vi "genIOL_Insertion.vi"(11 "Arm ID Ind":i32) -> (0 "zVisTraj":dbl[](array[numeric]) format="%_6g", 1 "yVisTraj":dbl[](array[numeric]) format="%_6g", 2 "xVisTraj":dbl[](array[numeric]) format="%_6g")   [LabVIEW 2016]
uses:
  <vilib>/Math Plots/3D Math Plots/3D Scatter/3D Scatter XCtrl/3D Scatter.xctl
  <vilib>/Math Plots/3D Math Plots/3D Scatter/3D Scatter Datatype/Public/Plot Helper (Vector).vi
  <vilib>/Analysis/NI_AALBase.lvlib
  <vilib>/Analysis/1siggen.llb/Ramp Pattern by Samples.vi
  <vilib>/gmath/NI_Gmath.lvlib
  Subsystems/Global Variables.vi
  <vilib>/Math Plots/3D Math Plots/3D Scatter/3D Scatter Datatype/3D Scatter Datatype.lvclass
panel:
  out "traj operational space":dbl[][](array[numeric])
  out "ind2":dbl
  out "ind1":dbl
  out "joint angles":dbl[][](array[numeric])
  in  "index":i32=200
  in  "PC path":path=path "D:/IRISSoft LV2016 beta/Host Demo/ThorlabsData/Eye1/VSCAN_0003.raw"
  in  "Iris path":path=path "D:/IRISSoft LV2016 beta/Host Demo/ThorlabsData/Eye1/VSCAN_0002.raw"
  out "Incision point":dbl[](array[numeric])
  out "Implement Injection Plot":refnum<class "3D Plot Datatype.lvclass">[](xcontrol)
  out "Implement joint angles":dbl[][](graph)
  out "min dist":dbl
  out "Actual Injection Plot":refnum<class "3D Plot Datatype.lvclass">[](xcontrol)
  out "End manual joint":dbl[](array[numeric])
  out "Start manual joint":dbl[](array[numeric])
  out "Planed joint angles":dbl[][](graph)
  out "Whole joint angles":dbl[][](graph)
  out "traj":dbl[][](array[numeric])
  out "ind":dbl
  out "Offset":dbl[][](array[numeric])
  out "Incision point index":dbl
  out "Planed Injection Plot":refnum<class "3D Plot Datatype.lvclass">[](xcontrol)
  out "current loop #":dbl
  out "x coordinates size 3":dbl
  out "x coordinates size 2":dbl
  out "x coordinates size":dbl
  out "x coordinates":dbl[](array[numeric])
  out "z coordinates":dbl[](array[numeric]) format="%#_13g"
  out "y coordinates":dbl[](array[numeric]) format="%#_13g"
  out "x coodi 2nd":dbl[](array[numeric]) format="%#_13g"
  in  "Total Time":dbl=60.0
  in  "Tip out Posit":dbl[](array[numeric])=[0.0, 0.0, 0.0] caption="Position [mm]" format="%#.3f"
  in  "Cycle Time [sec]":dbl[](array[numeric])=[60.0, 90.0, 120.0]
  in  "Sampling Rate [Hz]":i32=1000
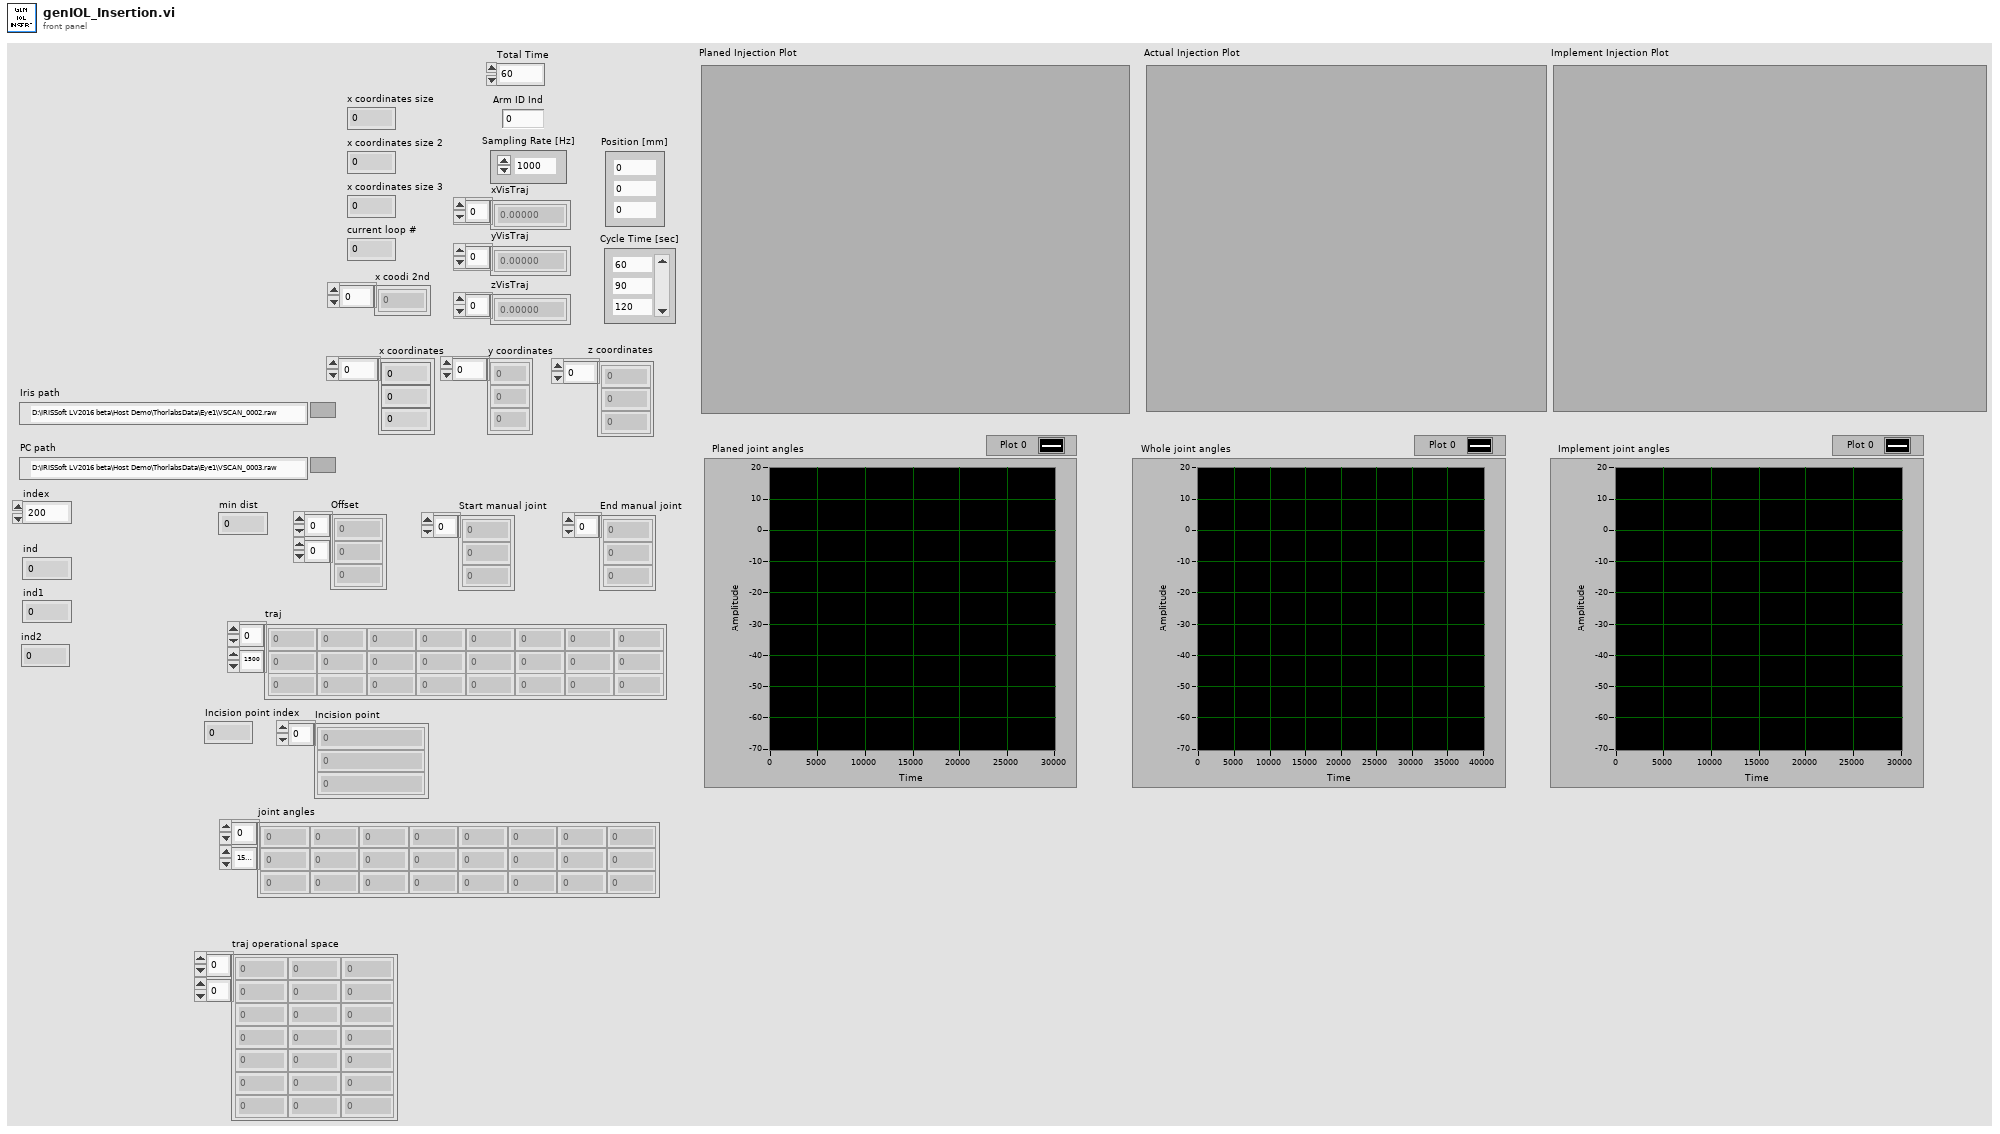
[diagram p1: front panel]
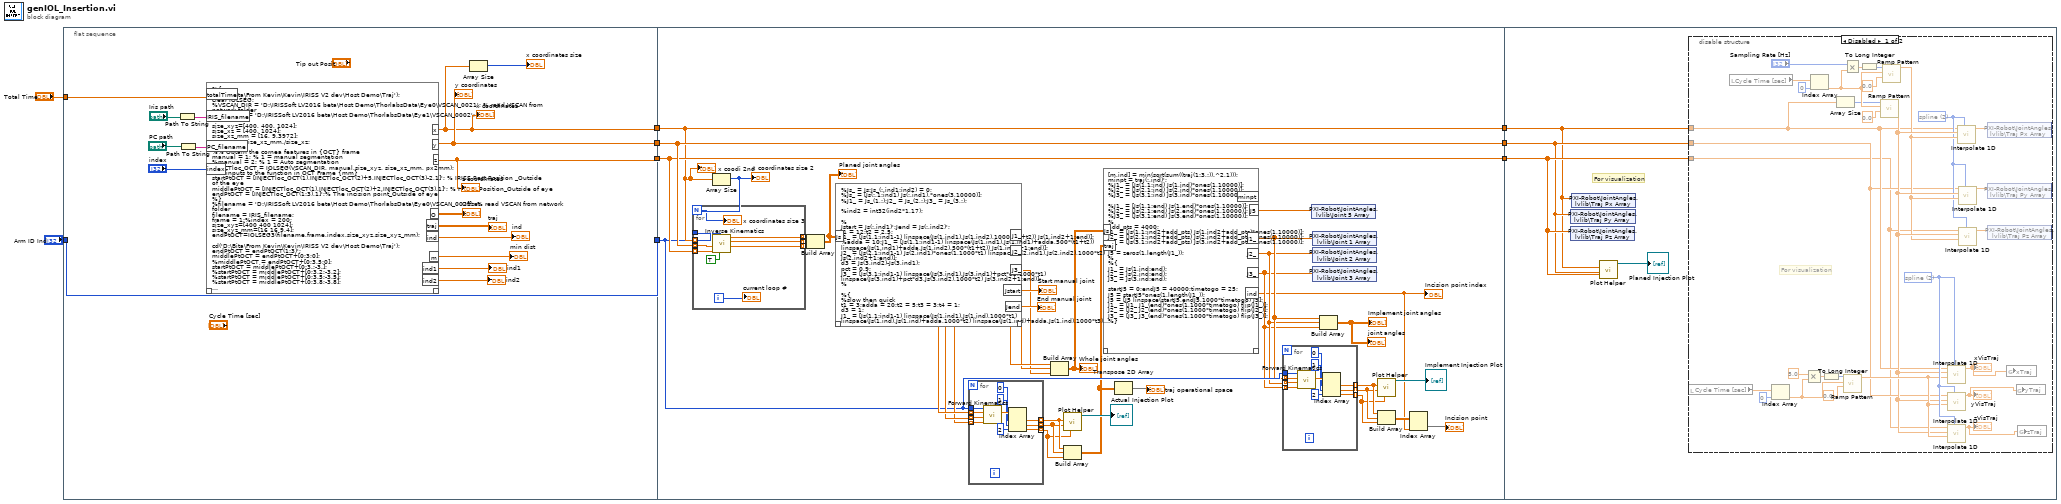
[diagram p0: block diagram]
diagram:
  n1 = flat-sequence {
    tunnel: "Arm ID Ind" -> [w26]
    tunnel: [w26] -> w8
    tunnel: [w22] -> w4
    tunnel: [w24] -> w3
    tunnel: [w23] -> w2
    tunnel: "Total Time" -> [w25]
    tunnel: w8 -> [w37]
    tunnel: [w57] -> w7
    tunnel: [w59] -> w6
    tunnel: [w58] -> w5
    tunnel: w4 -> [w57]
    tunnel: w3 -> [w59]
    tunnel: w2 -> [w58]
    tunnel: w7 -> [w92]
    tunnel: w6 -> [w93]
    tunnel: w5 -> [w94]
    frame #0 {
      n2 = Path To String(path="Iris path") -> (string=w15:string)
      n3 = Path To String(path="PC path") -> (string=w16:string)
      n4 = script code="%{\ncd('D:\\Bita\\From Kevin\\Kevin\\IRISS V2 dev\\Host Demo\\Traj');\nclear IOLSEG;\n%VSCAN_DIR = 'D:\\IRISSoft LV2016 beta\\Host Demo\\ThorlabsData\\Eye0\\VSCAN_0021'; % read VSCAN from network folder \nVSCAN_DIR = 'D:\\IRISSoft LV2016 beta\\Host Demo\\ThorlabsData\\Eye1\\VSCAN_0002';\n\nsize_xyz=[400, 400, 1024];\nsize_xz = [400, 1024]; \nsize_xz_mm = [16, 9.3972]; \npx2mm = size_xz_mm./size_xz; \n    \n%% Obtain the cornea features in {OCT} frame\nmanual = 1; % 1 = manual segmentation\n%manual = 2; % 1 = Auto segmentation\nINJECTloc_OCT = IOLSEG(VSCAN_DIR, manual,size_xyz, size_xz_mm, px2mm);\n%% inputs to the function in OCT Frame {mm}\nstartPtOCT = [INJECTloc_OCT(1),INJECTloc_OCT(2)+5,INJECTloc_OCT(3)-2,1]'; % IRISS Rest Position _Outside of the eye\nmiddlePtOCT = [INJECTloc_OCT(1),INJECTloc_OCT(2)+2,INJECTloc_OCT(3),1]'; % Home Position_Outside of eye\nendPtOCT = [INJECTloc_OCT(1:3),1]';% The incision point_Outside of eye\n%}\n%filename = 'D:\\IRISSoft LV2016 beta\\Host Demo\\ThorlabsData\\Eye0\\VSCAN_0021'; % read VSCAN from network folder \nfilename = IRIS_filename;\nframe = 1;%index = 200;\nsize_xyz=[400 400 1024];\nsize_xyz_mm=[16 16 9.4];\nendPtOCT=IOLSEG3(filename,frame,index,size_xyz,size_xyz_mm);\n\ncd('D:\\Bita\\From Kevin\\Kevin\\IRISS V2 dev\\Host Demo\\Traj');\nendPtOCT = endPtOCT(1:3)';\nmiddlePtOCT = endPtOCT+[0;3;0];\n%middlePtOCT = endPtOCT+[0;3.5;0];\nstartPtOCT = middlePtOCT+[0;3.;-3.];\n%startPtOCT = middlePtOCT+[0;3.2;-3.2];\n%startPtOCT = middlePtOCT+[0;3.5;-3.5];\n%startPtOCT = middlePtOCT+[0;3.8;-3.8];\n\n%middlePtOCT = endPtOCT+[0;-3;0];\n%startPtOCT = middlePtOCT+[0;-3.8;-3.8];\n\n%IRIS_filename = 'D:\\IRISSoft LV2016 beta\\Host Demo\\ThorlabsData\\Eye0\\VSCAN_0021.raw';\n%PC_filename = 'D:\\IRISSoft LV2016 beta\\Host Demo\\ThorlabsData\\Eye0\\VSCAN_0022.raw';\n%OCT_offset = 7; %OCT_offset = 0;\n%IRIS_filename = 'D:\\IRISSoft LV2016 beta\\Host Demo\\ThorlabsData\\Eye1\\VSCAN_0002.raw';\n%PC_filename = 'D:\\IRISSoft LV2016 beta\\Host Demo\\ThorlabsData\\Eye1\\VSCAN_0003.raw';\nOCT_offset = 13;\nspeed_scaler = 0.15;\n[tts,traj2,ind1,ind2]=IOL_injection_trajectory(startPtOCT,middlePtOCT,endPtOCT,IRIS_filename,PC_filename,OCT_offset,speed_scaler);\nTOI_file= 'D:\\IRISSoft LV2016 beta\\Host Demo\\TOI_static';\nfid_TOI = fopen(TOI_file,'r');\nTOI=fscanf(fid_TOI,'%f');\nTOI= reshape(TOI, [4 4])';\nfclose(fid_TOI);\n\nO = inv(TOI)*[endPtOCT;1];\n%{\ninit_X = 40;init_Y = 55;init_Z = 100;\ntime_to_go = norm(O(1:3))/.5;\nstage_X = linspace(init_X,init_X+O(1),1000*time_to_go);\nstage_Y = linspace(init_Y,init_Y+O(2),1000*time_to_go);\nstage_Z = linspace(init_Z,init_Z+O(3),1000*time_to_go);\n%}\n\nTOI2 = inv(TOI);TOI2(1:3,4) = TOI2(1:3,4)-O(1:3);\ntraj = TOI2*[traj2;ones(1,size(traj2,2))];\n%{\nTOI2_file= 'D:\\IRISSoft LV2016 beta\\Host Demo\\new_TOI.txt'\nfid_TOI2 = fopen(TOI2_file,'r');\nTOI2=fscanf(fid_TOI2,'%f');\nTOI2= reshape(TOI2, [4 4]);\nfclose(fid_TOI2);\ntraj = inv(TOI2)*[traj2;ones(1,size(traj2,2))];\n%}\n\nx = traj(1,:);y = traj(2,:);z = traj(3,:);\n[m,ind] = min(sqrt(sum((traj(1:3,:)).^2,1)));"("totalTime"=w25, "IRIS_filename"=w15, "PC_filename"=w16, "index"="index") -> ("x"=w22:dbl[], "y"=w24:dbl[], "z"=w23:dbl[], "O"=→"Offset":dbl[][], "ind"=→"ind":dbl, "traj"=→"traj":dbl[][], "ind1"=→"ind1":dbl, "ind2"=→"ind2":dbl, "m"=→"min dist":dbl)  [unwired: 1 in, 1 out]
      "y coordinates" <- w24
      "z coordinates" <- w23
      "x coordinates" <- w22
      n5 = Array Size(array=w22) -> (size(s)=→"x coordinates size":i32)
    }
    frame #1 {
      n6 = Array Size(array=w57) -> (size(s)=w56:i32)
      "x coordinates size 2" <- w56
      n7 = for {
        N: w56 -> [w86]
        tunnel: w37 -> [w87]
        tunnel: w57 -> [w91] mode=indexing
        tunnel: w59 -> [w90] mode=indexing
        tunnel: w58 -> [w89] mode=indexing
        tunnel: [w84] -> w54 mode=indexing
        tunnel: [w83] -> w53 mode=indexing
        tunnel: [w82] -> w55 mode=indexing
        i -> [w85]
        n8 = call "Inverse Kinematics.vi"("isToolTipInsideEye"=TRUE, "armID"=w87, "z"=w89, "y"=w90, "x"=w91) -> ("j3"=w83:dbl, "j2"=w84:dbl, "j1"=w82:dbl)  [unwired: 3 in, 1 out]
        "x coordinates size 3" <- w86
        "current loop #" <- w85
      }
      n9 = Build Array(w55, w54, w53) -> (w52:dbl[][])
      "Planed joint angles" <- w52
      n10 = script code="%Js_ = Js;Js_(:,ind1:ind2) = 0;\n%Js_ = [Js(:,1:ind1) Js(:,ind1).*ones(3,10000)];\n%J1_ = Js_(1,:);J2_ = Js_(2,:);J3_ = Js_(3,:);\n\n%ind2 = int32(ind2*1.17);\n\n%\nJstart = Js(:,ind1)';Jend = Js(:,ind2)';\nt1 = 12;t2 = 2.5;\nJ1_ = [Js(1,1:ind1-1) linspace(Js(1,ind1),Js(1,ind2),1000*(t1+t2)) Js(1,ind2+1:end)];\n%adda = 10;J1_ = [Js(1,1:ind1-1) linspace(Js(1,ind1),Js(1,ind1)+adda,500*(t1+t2)) linspace(Js(1,ind1)+adda,Js(1,ind2),500*(t1+t2)) Js(1,ind2+1:end)];\nJ2_ = [Js(2,1:ind1-1) Js(2,ind1)*ones(1,1000*t1) linspace(Js(2,ind1),Js(2,ind2),1000*t2) Js(2,ind2+1:end)];\nd3 = Js(3,ind2)-Js(3,ind1);\npct = 0.9;\nJ3_ = [Js(3,1:ind1-1) linspace(Js(3,ind1),Js(3,ind1)+pct*d3,1000*t1) linspace(Js(3,ind1)+pct*d3,Js(3,ind2),1000*t2) Js(3,ind2+1:end)];\n%\n\n%{\n%slow then quick\nt1 = 3;adda = 20;t2 = 5;t3 = 3;t4 = 1;\nd3 = 1;\nJ1_ = [Js(1,1:ind1-1) linspace(Js(1,ind1),Js(1,ind),1000*t1) linspace(Js(1,ind),Js(1,ind)+adda,1000*t2) linspace(Js(1,ind)+adda,Js(1,ind),1000*t3) linspace(Js(1,ind),Js(1,ind2),1000*t4)];\nJ2_ = [Js(2,1:ind1-1) linspace(Js(2,ind1),Js(2,ind),1000*t1) Js(2,ind)*ones(1,1000*(t2+t3)) linspace(Js(2,ind),Js(2,ind2),1000*t4)];\nJ3_ = [Js(3,1:ind1-1) linspace(Js(3,ind1),Js(3,ind),1000*t1) linspace(Js(3,ind),Js(3,ind)+d3,1000*t2) (Js(3,ind)+d3)*ones(1,1000*t3) linspace(Js(3,ind)+d3,Js(3,ind2),1000*t4)];\nlim_angle1 = -65;\nJ1_ = max(J1_,lim_angle1);\n%}\n%J1_ = [J1_(1:ind) J1_(ind)*ones(1,10000)];\n%J2_ = [J2_(1:ind) J2_(ind)*ones(1,10000)];\n%J3_ = [J3_(1:ind) J3_(ind)*ones(1,10000)];\n\n%startJ5 = 0;endJ5 = 40000;timetogo = 25;\n%J5 = startJ5*ones(1,length(J1_));\n%J5 = [J5 linspace(startJ5,endJ5,1000*timetogo) J5];\n%J1_ = [J1_ J1_(end)*ones(1,1000*timetogo) flip(J1_)];\n%J2_ = [J2_ J2_(end)*ones(1,1000*timetogo) flip(J2_)];\n%J3_ = [J3_ J3_(end)*ones(1,1000*timetogo) flip(J3_)];"("Js"=w52) -> ("J1_"=w49:dbl[], "J2_"=w48:dbl[], "J3_"=w47:dbl[], "Jstart"=→"Start manual joint":dbl[], "Jend"=→"End manual joint":dbl[])  [unwired: 1 in, 1 out]
      n11 = for {
        tunnel: w37 -> [w81]
        tunnel: w49 -> [w80] mode=indexing
        tunnel: w48 -> [w79] mode=indexing
        tunnel: w47 -> [w78] mode=indexing
        tunnel: [w73] -> w45 mode=indexing
        tunnel: [w72] -> w44 mode=indexing
        tunnel: [w71] -> w43 mode=indexing
        n12 = call "Forward Kinematics.vi"("j3"=w78, "j2"=w79, "j1"=w80, "armID"=w81) -> ("XYZ Out Array"=w77:dbl[])  [unwired: 7 in]
        n13 = Index Array(array=w77, index #1=0 ("index"), index #2=1 ("index"), index #3=2 ("index")) -> (element #1=w73:dbl, element #2=w72:dbl, element #3=w71:dbl)
      }
      n14 = Build Array(w49, w48, w47) -> (w36:dbl[][])
      "Whole joint angles" <- w36
      n15 = call-poly <vilib>:"Plot Helper.vi"("z vector"=w43, "y vector"=w44, "x vector"=w45) -> ("3D Plot lvclass Array out"=→"Actual Injection Plot":refnum<class "3D Plot Datatype.lvclass">[])  [unwired: 3 in, 5 out]
      n16 = Build Array(w45, w44, w43) -> (w27:dbl[][])
      n17 = script code="[m,ind] = min(sqrt(sum((traj(1:3,:)).^2,1)));\nminpt = traj(:,ind)';\n%J1_ = [Js(1,1:ind) Js(1,ind)*ones(1,10000)];\n%J2_ = [Js(2,1:ind) Js(2,ind)*ones(1,10000)];\n%J3_ = [Js(3,1:ind) Js(3,ind)*ones(1,10000)];\n\n%J1_ = [Js(1,1:end) Js(1,end)*ones(1,10000)];\n%J2_ = [Js(2,1:end) Js(2,end)*ones(1,10000)];\n%J3_ = [Js(3,1:end) Js(3,end)*ones(1,10000)];\n%\nadd_pts = 4000;\nJ1_ = [Js(1,1:ind2+add_pts) Js(1,ind2+add_pts)*ones(1,10000)];\nJ2_ = [Js(2,1:ind2+add_pts) Js(2,ind2+add_pts)*ones(1,10000)];\nJ3_ = [Js(3,1:ind2+add_pts) Js(3,ind2+add_pts)*ones(1,10000)];\n\nJ5 = zeros(1,length(J1_));\n%\n%{\nJ1_ = Js(1,ind:end);\nJ2_ = Js(2,ind:end);\nJ3_ = Js(3,ind:end);\n\nstartJ5 = 0;endJ5 = 40000;timetogo = 25;\nJ5 = startJ5*ones(1,length(J1_));\nJ5 = [J5 linspace(startJ5,endJ5,1000*timetogo) J5];\nJ1_ = [J1_ J1_(end)*ones(1,1000*timetogo) flip(J1_)];\nJ2_ = [J2_ J2_(end)*ones(1,1000*timetogo) flip(J2_)];\nJ3_ = [J3_ J3_(end)*ones(1,1000*timetogo) flip(J3_)];\n%}"("Js"=w36, "traj"=w27) -> ("J1_"=w35:dbl[], "J2_"=w34:dbl[], "J3_"=w33:dbl[], "ind"=w31:dbl, "J5"=w38:dbl[])  [unwired: 1 in, 2 out]
      "Incision point index" <- w31
      n18 = Transpose 2D Array(2D array=w27) -> (transposed array=→"traj operational space":dbl[][])
      n19 = for {
        tunnel: w37 -> [w70]
        tunnel: w35 -> [w69] mode=indexing
        tunnel: w34 -> [w68] mode=indexing
        tunnel: w33 -> [w67] mode=indexing
        tunnel: [w62] -> w41 mode=indexing
        tunnel: [w61] -> w40 mode=indexing
        tunnel: [w60] -> w39 mode=indexing
        n20 = call "Forward Kinematics.vi"("j3"=w67, "j2"=w68, "j1"=w69, "armID"=w70) -> ("XYZ Out Array"=w66:dbl[])  [unwired: 7 in]
        n21 = Index Array(array=w66, index #1=0 ("index"), index #2=1 ("index"), index #3=2 ("index")) -> (element #1=w62:dbl, element #2=w61:dbl, element #3=w60:dbl)
      }
      n22 = shared-variable "PXI-Robot\\JointAngles.lvlib\\Joint 5 Array"(w38) -> ()  [unwired: 1 in, 1 out]
      n23 = shared-variable "PXI-Robot\\JointAngles.lvlib\\Joint 1 Array"(w35) -> ()  [unwired: 1 in, 1 out]
      n24 = shared-variable "PXI-Robot\\JointAngles.lvlib\\Joint 2 Array"(w34) -> ()  [unwired: 1 in, 1 out]
      n25 = shared-variable "PXI-Robot\\JointAngles.lvlib\\Joint 3 Array"(w33) -> ()  [unwired: 1 in, 1 out]
      n26 = Build Array(w35, w34, w33) -> (→"Implement joint angles" →"joint angles":dbl[][])
      n27 = call-poly <vilib>:"Plot Helper.vi"("z vector"=w39, "y vector"=w40, "x vector"=w41) -> ("3D Plot lvclass Array out"=→"Implement Injection Plot":refnum<class "3D Plot Datatype.lvclass">[])  [unwired: 3 in, 5 out]
      n28 = Build Array(w41, w40, w39) -> (w32:dbl[][])
      n29 = Index Array(array=w32, index (col)=w31) -> (element=→"Incision point":dbl[])  [unwired: 1 in]
      "x coodi 2nd" <- w57
    }
    frame #2 {
      # "For visualization"
      n30 = shared-variable "PXI-Robot\\JointAngles.lvlib\\Traj Py Array"(w93) -> ()  [unwired: 1 in, 1 out]
      n31 = shared-variable "PXI-Robot\\JointAngles.lvlib\\Traj Pz Array"(w94) -> ()  [unwired: 1 in, 1 out]
      n32 = shared-variable "PXI-Robot\\JointAngles.lvlib\\Traj Px Array"(w92) -> ()  [unwired: 1 in, 1 out]
      n33 = call-poly <vilib>:"Plot Helper.vi"("z vector"=w94, "y vector"=w93, "x vector"=w92) -> ("3D Plot lvclass Array out"=→"Planed Injection Plot":refnum<class "3D Plot Datatype.lvclass">[])  [unwired: 3 in, 5 out]
      n34 = disable-structure shown="Disabled" {
        disable-tunnel: w92 -> [w101 _]
        disable-tunnel: w93 -> [w100 _]
        disable-tunnel: w94 -> [w99 _]
        frame Disabled {
          w113 = 2 items=["nearest", "linear", "spline", "cubic Hermite", "Lagrange"] ("method")
          w102 = 2 items=["nearest", "linear", "spline", "cubic Hermite", "Lagrange"] ("method")
          # "For visualization"
          n35 = local read "Cycle Time [sec]"() -> (w107:dbl[])
          n36 = local read "Cycle Time [sec]"() -> (w125:dbl[])
          n37 = Index Array(array=w107, index=0) -> (element=w108:dbl)
          n38 = Multiply(x=5.0, y=w108) -> (x*y=w110:dbl)
          n39 = Index Array(array=w125, index=0) -> (element=w118:dbl)
          n40 = To Long Integer(number=w110) -> (32bit integer=w111:i32)
          n41 = Array Size(array=w101) -> (size(s)=w117:i32)
          n42 = call-poly <vilib>:"Ramp Pattern.vi"("start"=0.0, "end"=w108, "samples"=w111) -> ("Ramp Pattern"=w105:dbl[])  [unwired: 7 in, 1 out]
          n43 = Multiply(x="Sampling Rate [Hz]", y=w118) -> (x*y=w121:dbl)
          n44 = To Long Integer(number=w121) -> (32bit integer=w122:i32)
          n45 = call-poly <vilib>:"Ramp Pattern.vi"("start"=0.0, "end"=w118, "samples"=w117) -> ("Ramp Pattern"=w104:dbl[])  [unwired: 7 in, 1 out]
          n46 = call-poly <vilib>:"Ramp Pattern.vi"("start"=0.0, "end"=w118, "samples"=w122) -> ("Ramp Pattern"=w103:dbl[])  [unwired: 7 in, 1 out]
          n47 = call <vilib>:"Interpolate 1D.vi"("method"=w113, "xi"=w105, "X"=w104, "Y"=w101) -> ("yi"=w96:dbl[])  [unwired: 5 in, 2 out]
          "xVisTraj" <- w96
          n48 = call <vilib>:"Interpolate 1D.vi"("method"=w113, "xi"=w105, "X"=w104, "Y"=w100) -> ("yi"=w97:dbl[])  [unwired: 5 in, 2 out]
          "yVisTraj" <- w97
          n49 = call <vilib>:"Interpolate 1D.vi"("method"=w113, "xi"=w105, "X"=w104, "Y"=w99) -> ("yi"=w98:dbl[])  [unwired: 5 in, 2 out]
          "zVisTraj" <- w98
          n50 = call <vilib>:"Interpolate 1D.vi"("method"=w102, "xi"=w103, "X"=w104, "Y"=w101) -> ("yi"=w115:dbl[])  [unwired: 5 in, 2 out]
          n51 = call <vilib>:"Interpolate 1D.vi"("method"=w102, "xi"=w103, "X"=w104, "Y"=w100) -> ("yi"=w116:dbl[])  [unwired: 5 in, 2 out]
          n52 = call <vilib>:"Interpolate 1D.vi"("method"=w102, "xi"=w103, "X"=w104, "Y"=w99) -> ("yi"=w114:dbl[])  [unwired: 5 in, 2 out]
          n53 = shared-variable "PXI-Robot\\JointAngles.lvlib\\Traj Px Array"(w115) -> ()  [unwired: 1 in, 1 out]
          n54 = shared-variable "PXI-Robot\\JointAngles.lvlib\\Traj Py Array"(w116) -> ()  [unwired: 1 in, 1 out]
          n55 = shared-variable "PXI-Robot\\JointAngles.lvlib\\Traj Pz Array"(w114) -> ()  [unwired: 1 in, 1 out]
          n56 = global write "Global Variables.vi" "xTraj"(w96) -> ()
          n57 = global write "Global Variables.vi" "yTraj"(w97) -> ()
          n58 = global write "Global Variables.vi" "zTraj"(w98) -> ()
        }
        frame Enabled {
        }
      }
    }
  }
